vi "Hightlight.vi"(8 "error in (no error)":errorcluster, 10 "Table in":refnum<vi>, 11 "State":T1={"logTable"=refnum, "max items"=500, "displaydata"=[], "data"=[], "Auto Scroll"=TRUE, "current item"=500, "col headers"=[], "Add to Top"=TRUE, "Auto resize"=TRUE, "col size"=[], "filters"=[], "color cells"=[]}) -> (0 "error out":errorcluster, 2 "Table out":refnum<vi>, 3 "State (dup)":T1={"logTable"=refnum, "max items"=500, "displaydata"=[], "data"=[], "Auto Scroll"=TRUE, "current item"=500, "col headers"=[], "Add to Top"=TRUE, "Auto resize"=TRUE, "col size"=[], "filters"=[], "color cells"=[]})   [LabVIEW 2013, in "UI-DisplayTable(dev).xctl"]
uses:
  UI-DisplayTable(dev).xctl
  State.ctl
  DEF-Filter.ctl
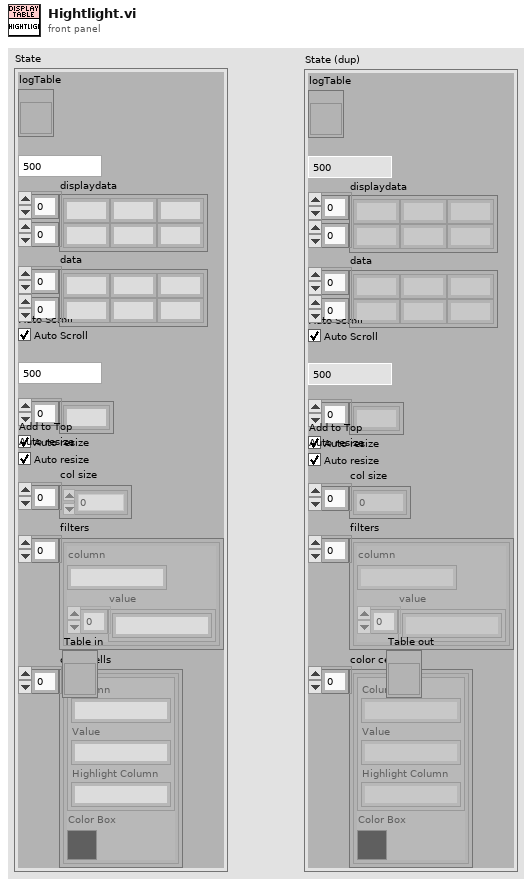
[diagram p1: front panel]
types:
  T1 = typedef "UI-DisplayTable(dev).xctl/State.ctl" = cluster{"logTable":refnum<vi>, "max items":i32, "displaydata":string[][], "data":string[][], "Auto Scroll":bool, "current item":i32, "col headers":string[], "Add to Top":bool, "Auto resize":bool, "col size":i32[], "filters":T2[], "color cells":cluster{"color cell":cluster{"Column":string, "Value":string, "Highlight Column":string}, "Color Box":u32}[]}
  T2 = typedef "UI-DisplayTable(dev).xctl/DEF-Filter.ctl" = cluster{"column":string, "value":string[]}
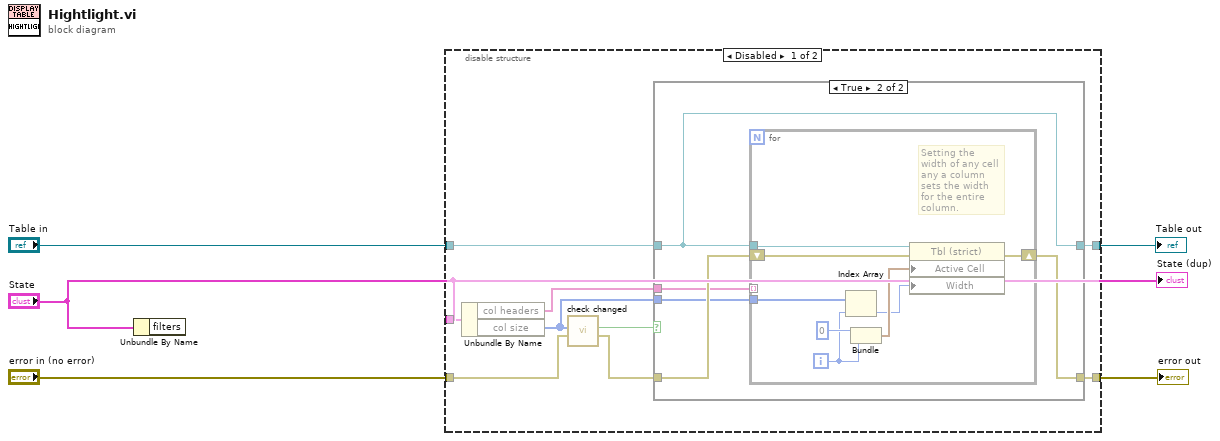
[diagram p0: block diagram]
diagram:
  n1 = Unbundle By Name("State") -> ()  [unwired: 1 out]
  n2 = disable-structure shown="Disabled" {
    disable-tunnel: "State" -> [w14 _]
    disable-tunnel: "Table in" -> [w11 w31]
    disable-tunnel: [w10 w31] -> w4
    disable-tunnel: "error in (no error)" -> [w9 w30]
    disable-tunnel: [w7 w30] -> w1
    frame Disabled {
      n3 = Unbundle By Name(w14) -> ("col headers"=w6:string[], "col size"=w12:i32[])
      n4 = call "check changed.vi"("error in (no error)"=w9, "data"=w12) -> ("error out"=w8:errorcluster, "changed?"=w13:bool)  [unwired: 8 in]
      n5 = case shown="True" w13 {
        tunnel: w12 -> [_ w18]
        tunnel: w11 -> [w16 w21]
        tunnel: [w16 w21] -> w10
        tunnel: w8 -> [w15 w20]
        tunnel: [w15 w19] -> w7
        tunnel: w6 -> [_ w17]
        frame False {
        }
        frame True {
          n6 = for {
            tunnel: w21 -> [w28]
            shift-right: [w26] -> w19
            shift-left: w20 -> [w27]
            tunnel: w18 -> [w24]
            tunnel: w17 -> [_] mode=indexing
            i -> [w23]
            # "Setting the width of any cell any a column sets the width for the entire column."
            n7 = Index Array(array=w24, index=w23) -> (element=w22:i32)
            n8 = Bundle(0, w23) -> (w29:cluster{i32, i32})  [unwired: 1 in]
            n9 = property class="Tbl (strict)"(reference=w28, error in=w27, "Active Cell"=w29, "Width"=w22) -> (error out=w26:errorcluster)  [unwired: 1 out]
          }
        }
      }
    }
    frame Enabled {
    }
  }
  "error out" <- w1
  "Table out" <- w4
  "State (dup)" <- "State"
